vi "Parse Tree Labels.vi"(5 "FIFO Idx Qs":T1, 6 "Channel handle in":u32, 7 "Access":T2, 8 "error out":errorcluster, 10 "Label Refs":T3[](array[typedef]) format="%.0x", 11 "Custom Device Ref":T3 format="%.0x") -> (0 "error out":errorcluster, 1 "Transfer Periods":u32[](array[numeric]), 2 "Label Map":i32[](array[numeric]), 3 "Label data":T4[](array[typedef]) {"Words"."Param Setting"."Num Bits" min=1 max=32; "Words"."Param Setting"."Start Bit" min=8 max=31; "Words"."Block Data Refs"."Data Reference" format="%.0x"; "Label" format="%.0o"})   [LabVIEW 2012, in "AIT 429 Engine.lvlib"]
uses:
  AIT 429 Engine.lvlib
  <vilib>/NI Veristand/Custom Device API/Custom Device Item Ref.ctl
  RT Controls/RT Label Settings.ctl
  Shared/Controls and Global/Label.ctl
  Shared/Controls and Global/transferPeriod.ctl
  RT Controls/Driver Data.ctl
  RT Controls/RT Word Settings.ctl
  <vilib>/NI Veristand/Custom Device API/Block Data Reference.ctl
  <vilib>/NI Veristand/Custom Device API/Data Reference.ctl
  RT Controls/RT Param Setting.ctl
  Shared/Controls and Global/Start Bit.ctl
  Shared/Controls and Global/Number of Bits.ctl
  Shared/Controls and Global/TransferType.ctl
  <vilib>/NI Veristand/Custom Device API/Data Access Type.ctl
  RT Controls/FIFO Idx Qs.ctl
  RT Controls/Data Ref FGV Command.ctl
  Shared/Controls and Global/Global.vi
  <vilib>/NI Veristand/Custom Device Tools/Custom Device Utility Library/NI VeriStand - Search for All Items by GUID.vi
  <vilib>/NI Veristand/Custom Device Tools/Custom Device Utility Library/NI VeriStand - Search for Item by GUID.vi
  <vilib>/NI Veristand/Custom Device API/Get Item Property (U16).vi
  <vilib>/NI Veristand/Custom Device API/Get Item Property (U32).vi
  <vilib>/NI Veristand/Custom Device API/Get Item Property (String).vi
  <vilib>/NI Veristand/Custom Device API/Get Item Property (Boolean).vi
  <vilib>/NI Veristand/Custom Device API/Get Item Property (Double).vi
  <vilib>/NI Veristand/Custom Device API/Get Item Property (I32).vi
  ARINC 429 Shared.lvlib
  <vilib>/NI Veristand/Custom Device API/Custom Device API.lvlib
  <vilib>/NI Veristand/Custom Device Tools/Custom Device Utility Library/Custom Device Utility Library.lvlib
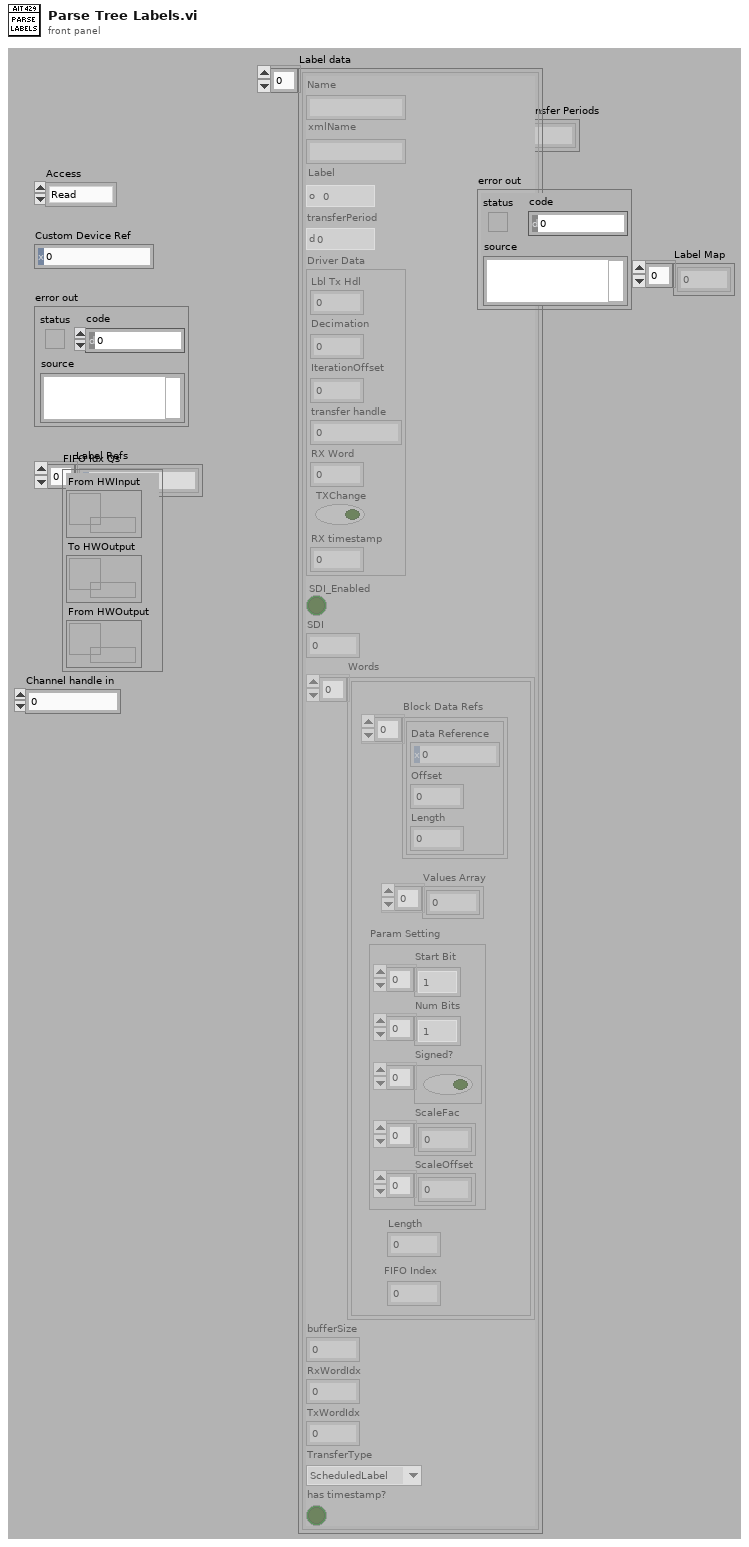
[diagram p1: front panel]
types:
  T1 = typedef "AIT 429 Engine.lvlib/FIFO Idx Qs.ctl" = cluster{"From HWInput":refnum<queue>, "To HWOutput":refnum<queue>, "From HWOutput":refnum<queue>}
  T2 = typedef "Custom Device API.lvlib/Data Access Type.ctl" = enum16{"Read", "Write"}
  T3 = typedef "Custom Device API.lvlib/Custom Device Item Ref.ctl" = u64
  T4 = typedef "AIT 429 Engine.lvlib/RT Label Settings.ctl" = cluster{"Name":string, "xmlName":string, "Label":T5, "transferPeriod":T6, "Driver Data":T7, "SDI_Enabled":bool, "SDI":u8, "Words":T8[], "bufferSize":u32, "RxWordIdx":i32, "TxWordIdx":i32, "TransferType":T14, "has timestamp?":bool}
  T5 = typedef "ARINC 429 Shared.lvlib/Label.ctl" = u8
  T6 = typedef "ARINC 429 Shared.lvlib/transferPeriod.ctl" = u32
  T7 = typedef "AIT 429 Engine.lvlib/Driver Data.ctl" = cluster{"Lbl Tx Hdl":u32, "Decimation":i32, "IterationOffset":i32, "transfer handle":u32, "RX Word":u32, "TXChange":bool, "RX timestamp":dbl}
  T8 = typedef "AIT 429 Engine.lvlib/RT Word Settings.ctl" = cluster{"Block Data Refs":T9[], "Values Array":dbl[], "Length":i32, "FIFO Index":i32, "Param Setting":T11}
  T9 = typedef "Custom Device API.lvlib/Block Data Reference.ctl" = cluster{"Data Reference":T10, "Offset":i32, "Length":i32}
  T10 = typedef "Custom Device API.lvlib/Data Reference.ctl" = i32
  T11 = typedef "AIT 429 Engine.lvlib/RT Param Setting.ctl" = cluster{"Start Bit":T12[], "Num Bits":T13[], "Signed?":bool[], "ScaleFac":dbl[], "ScaleOffset":dbl[]}
  T12 = typedef "ARINC 429 Shared.lvlib/Start Bit.ctl" = i32
  T13 = typedef "ARINC 429 Shared.lvlib/Number of Bits.ctl" = i32
  T14 = typedef "ARINC 429 Shared.lvlib/TransferType.ctl" = enum16{"ScheduledLabel", "Acyclic", "Block", "Strobe"}
  T15 = typedef "AIT 429 Engine.lvlib/Data Ref FGV Command.ctl" = enum16{"Intialize", "Get", "Update"}
  T16 = typedef "Custom Device API.lvlib/Custom Device Item Info.ctl" = cluster{"Name":string, "Is Channel":bool, "GUID":string, "Is Waveform":bool}
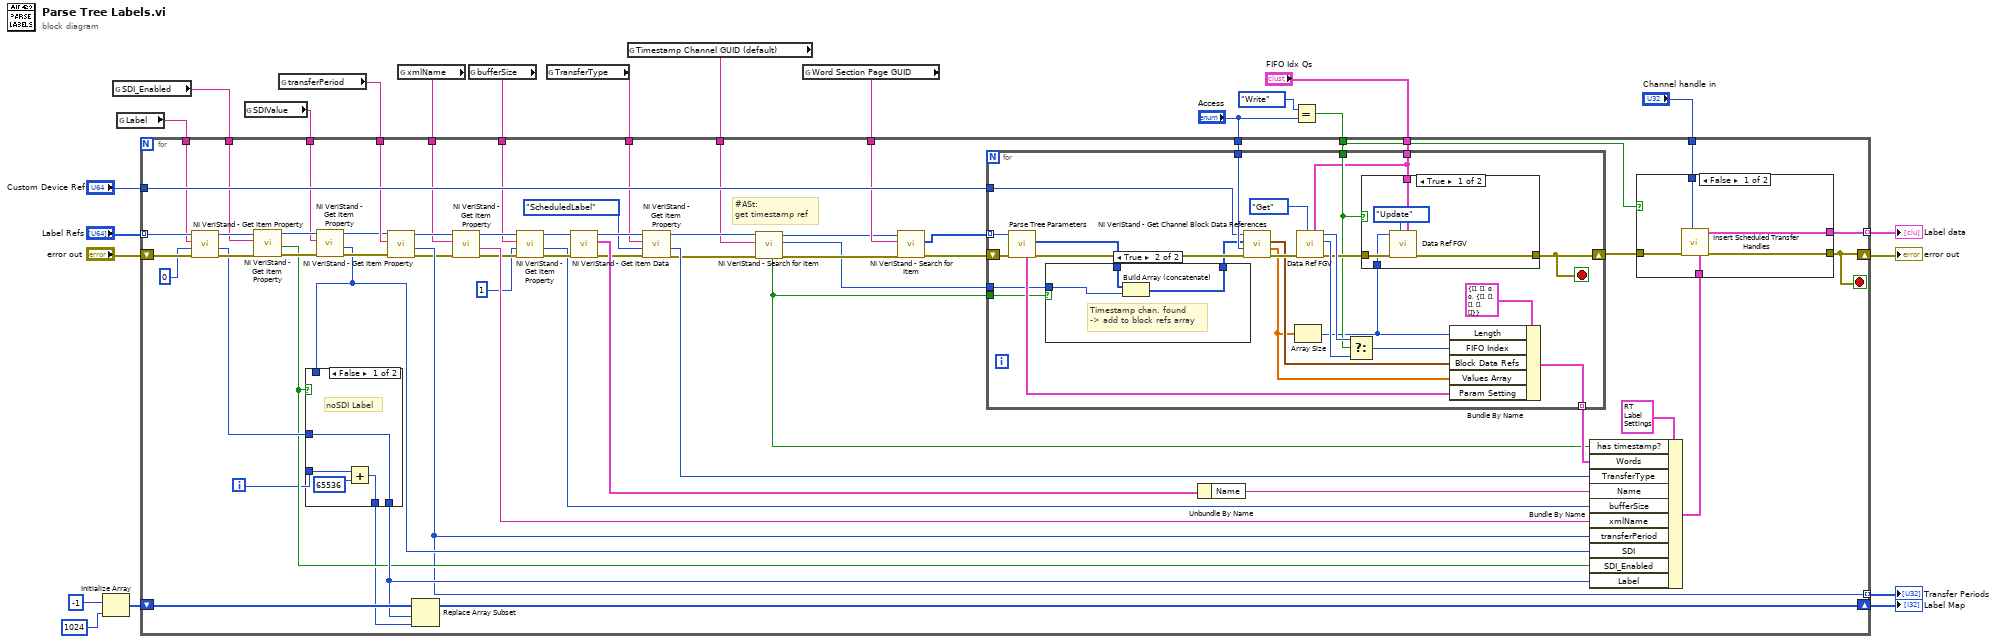
[diagram p0: block diagram]
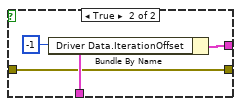
[diagram p2: hidden frame]
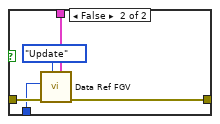
[diagram p4: hidden frame]
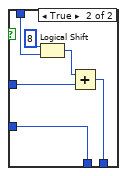
[diagram p5: hidden frame]
diagram:
  n1 = Initialize Array(-1 ("index"), 1024 ("dimension size")) -> (w14:i32[])
  n2 = global read "Global.vi" "SDI_Enabled"() -> (w8:string)
  n3 = global read "Global.vi" "Label"() -> (w12:string)
  n4 = global read "Global.vi" "SDIValue"() -> (w7:string)
  n5 = global read "Global.vi" "transferPeriod"() -> (w11:string)
  n6 = global read "Global.vi" "xmlName"() -> (w6:string)
  n7 = global read "Global.vi" "bufferSize"() -> (w5:string)
  n8 = global read "Global.vi" "TransferType"() -> (w2:string)
  n9 = global read "Global.vi" "Timestamp Channel GUID (default)"() -> (w1:string)
  n10 = global read "Global.vi" "Word Section Page GUID"() -> (w4:string)
  n11 = Equal?(x=Data_Access_Type."Write" ("y"), y="Access") -> (x = y?=w10:bool)
  n12 = for {
    tunnel: "Label Refs" -> [w85] mode=indexing
    shift-right: [w40] -> w20
    shift-left: "error out" -> [w81]
    tunnel: "Access" -> [w82]
    tunnel: "Custom Device Ref" -> [w77]
    tunnel: [w61] -> w24 mode=indexing
    tunnel: "FIFO Idx Qs" -> [w74]
    shift-right: [w78] -> w13
    shift-left: w14 -> [w79]
    tunnel: w12 -> [w76]
    tunnel: w11 -> [w75]
    tunnel: w10 -> [w45]
    tunnel: "Channel handle in" -> [w43]
    tunnel: w8 -> [w71]
    tunnel: w7 -> [w66]
    tunnel: w6 -> [w58]
    tunnel: w5 -> [w51]
    tunnel: w4 -> [w47]
    tunnel: [w41] -> w3 mode=indexing
    tunnel: w2 -> [w35]
    tunnel: w1 -> [w27]
    i -> [w56]
    stop <- w40 stop-if-true
    # "#ASt:\nget timestamp ref"
    n13 = call-poly <vilib>:"NI VeriStand - Get Item Property.vi"("error in (no error)"=w81, "Default Value"=T5 0 ("Label"), "Property Name"=w76, "Item Ref in"=w85) -> ("error out"=w72:errorcluster, "Value"=w65:u32, "Item Ref out"=w73:T3)  [unwired: 4 in, 1 out]
    n14 = call-poly <vilib>:"NI VeriStand - Get Item Property.vi"("error in (no error)"=w72, "Property Name"=w71, "Item Ref in"=w73) -> ("error out"=w68:errorcluster, "Value"=w63:bool, "Item Ref out"=w70:T3)  [unwired: 5 in, 1 out]
    n15 = call-poly <vilib>:"NI VeriStand - Get Item Property.vi"("error in (no error)"=w68, "Property Name"=w66, "Item Ref in"=w70) -> ("error out"=w67:errorcluster, "Value"=w62:u32, "Item Ref out"=w69:T3)  [unwired: 5 in, 1 out]
    n16 = case shown="False" w63 {
      tunnel: w62 -> [_ w142]
      tunnel: w65 -> [w136 w139]
      tunnel: [w136 w138] -> w64
      tunnel: w56 -> [w135 w137]
      tunnel: [w134 w137] -> w55
      frame False {
        # "noSDI Label"
        n17 = Add(x=w135, y=65536) -> (x+y=w134:i32)
      }
      frame True {
        n18 = Logical Shift(y=u32 8 ("x"), x=w142) -> (x << y=w140:u32)
        n19 = Add(x=w140, y=w139) -> (x+y=w138:u32)
      }
    }
    n20 = call-poly <vilib>:"NI VeriStand - Get Item Property.vi"("error in (no error)"=w67, "Property Name"=w75, "Item Ref in"=w69) -> ("error out"=w59:errorcluster, "Value"=w61:u32, "Item Ref out"=w60:T3)  [unwired: 5 in, 1 out]
    n21 = Replace Array Subset(array=w79, new element=w55, index=w64) -> (w78:i32[])
    n22 = call-poly <vilib>:"NI VeriStand - Get Item Property.vi"("error in (no error)"=w59, "Property Name"=w58, "Item Ref in"=w60) -> ("error out"=w54:errorcluster, "Value"=w57:string, "Item Ref out"=w52:T3)  [unwired: 5 in, 1 out]
    n23 = call-poly <vilib>:"NI VeriStand - Get Item Property.vi"("error in (no error)"=w54, "Default Value"=u32 1, "Property Name"=w51, "Item Ref in"=w52) -> ("error out"=w53:errorcluster, "Value"=w50:u32, "Item Ref out"=w49:T3)  [unwired: 4 in, 1 out]
    n24 = call <vilib>:"NI VeriStand - Get Item Data.vi"("error in (no error)"=w53, "Item Ref in"=w49) -> ("error out"=w36:errorcluster, "Item Info"=w83:T16, "Item Ref out"=w37:T3)  [unwired: 6 in, 1 out]
    n25 = call-poly <vilib>:"NI VeriStand - Get Item Property.vi"("error in (no error)"=w36, "Default Value"=TransferType."ScheduledLabel" ("TransferType"), "Property Name"=w35, "Item Ref in"=w37) -> ("error out"=w30:errorcluster, "Value"=w34:u16, "Item Ref out"=w31:T3)  [unwired: 4 in, 1 out]
    n26 = call-poly <vilib>:"NI VeriStand - Search for Item.vi"("error in"=w30, "Item GUID"=w27, "Section Ref in"=w31) -> ("error out"=w29:errorcluster, "Item Ref"=w26:T3, "Section Ref out"=w28:T3, "Found"=w25:bool)  [unwired: 5 in]
    n27 = call-poly <vilib>:"NI VeriStand - Search for Item.vi"("error in"=w29, "Item GUID"=w47, "Section Ref in"=w28) -> ("error out"=w48:errorcluster, "Item Refs"=w39:T3[])  [unwired: 5 in, 2 out]
    n28 = for {
      tunnel: w82 -> [w118]
      tunnel: w77 -> [w111]
      tunnel: w45 -> [w110]
      tunnel: w74 -> [w109]
      shift-right: [w107] -> w42
      shift-left: w48 -> [w108]
      tunnel: w39 -> [w106] mode=indexing
      tunnel: [w101] -> w46 mode=indexing
      tunnel: w25 -> [w97]
      tunnel: w26 -> [w98]
      stop <- w107 stop-if-true
      n29 = call "Parse Tree Parameters.vi"("error in"=w108, "Item Ref in"=w106) -> ("error out"=w117:errorcluster, "Parameter References"=w96:T3[], "Parameter Driver Data"=w104:T11)  [unwired: 6 in, 1 out]
      n30 = case shown="True" w97 {
        tunnel: w98 -> [_ w120]
        tunnel: w96 -> [w119 w122]
        tunnel: [w119 w121] -> w95
        frame False {
        }
        frame True {
          # "Timestamp chan. found\n-> add to block refs array"
          n31 = Build Array (concatenate)(w122, w120) -> (w121:T3[])
        }
      }
      n32 = call <vilib>:"NI VeriStand - Get Channel Block Data References.vi"("error in (no error)"=w117, "Access"=w118, "Channel Refs"=w95, "Device Ref in"=w111) -> ("error out"=w116:errorcluster, "Values Array"=w99:dbl[], "Block Data Refs"=w100:T9[])  [unwired: 4 in, 1 out]
      n33 = Array Size(array=w99) -> (size(s)=w102:i32)
      n34 = call "Data Ref FGV.vi"("FIFO Idx Qs"=w109, "Command"=Data_Ref_FGV_Command."Get", "error in (no error)"=w116) -> ("error out"=w112:errorcluster, "To HWOutput FIFO Index / Length"=w113:i32, "From HWInput FIFO Index / Length"=w114:i32)  [unwired: 5 in, 1 out]
      n35 = Select(t=w114, s=w110, f=w113) -> (s? t:f=w103:i32)
      n36 = case shown="True" w110 {
        tunnel: w112 -> [w127 w132]
        tunnel: [w124 w128] -> w107
        tunnel: w102 -> [w125 w130]
        tunnel: w109 -> [w123 w129]
        frame True {
          n37 = call "Data Ref FGV.vi"("FIFO Idx Qs"=w123, "Command"=Data_Ref_FGV_Command."Update", "error in (no error)"=w127, "From HWInput Length"=w125) -> ("error out"=w124:errorcluster)  [unwired: 4 in, 3 out]
        }
        frame False {
          n38 = call "Data Ref FGV.vi"("FIFO Idx Qs"=w129, "Command"=Data_Ref_FGV_Command."Update", "error in (no error)"=w132, "To HWOutput Length"=w130) -> ("error out"=w128:errorcluster)  [unwired: 4 in, 3 out]
        }
      }
      n39 = Bundle By Name(cluster=T8 {"Block Data Refs"=[], "Values Array"=[], "Length"=0, "FIFO Index"=0, "Param Setting"={"Start Bit"=[], "Num Bits"=[], "Signed?"=[], "ScaleFac"=[], "ScaleOffset"=[]}} ("Word"), "Length"=w102, "FIFO Index"=w103, "Block Data Refs"=w100, "Values Array"=w99, "Param Setting"=w104) -> (w101:T8)
    }
    n40 = Unbundle By Name(w83) -> ("Name"=w38:string)
    n41 = Bundle By Name(cluster=T4 {"Name"="", "xmlName"="", "Label"=0, "transferPeriod"=0, "Driver Data"={"Lbl Tx Hdl"=0, "Decimation"=0, "IterationOffset"=0, "transfer handle"=0, "RX Word"=0, "TXChange"=FALSE, "RX timestamp"=0.0}, "SDI_Enabled"=FALSE, "SDI"=0, "Words"=[], "bufferSize"=0, "RxWordIdx"=0, "TxWordIdx"=0, "TransferType"=enum."ScheduledLabel", "has timestamp?"=FALSE} ("Label"), "has timestamp?"=w25, "Words"=w46, "TransferType"=w34, "Name"=w38, "bufferSize"=w50, "xmlName"=w57, "transferPeriod"=w61, "SDI"=w62, "SDI_Enabled"=w63, "Label"=w64) -> (w44:T4)
    n42 = case shown="False" w45 {
      tunnel: w44 -> [w89 w94]
      tunnel: w43 -> [w90 _]
      tunnel: w42 -> [w88 w92]
      tunnel: [w87 w92] -> w40
      tunnel: [w86 w91] -> w41
      frame False {
        n43 = call "Insert Scheduled Transfer Handles.vi"("Label in"=w89, "Tx channel handle in"=w90, "error in (no error)"=w88) -> ("error out"=w87:errorcluster, "Label out"=w86:T4)  [unwired: 7 in]
      }
      frame True {
        n44 = Bundle By Name(cluster=w94, "Driver Data.IterationOffset"=-1) -> (w91:T4)
      }
    }
  }
  "Transfer Periods" <- w24
  "Label data" <- w3
  "error out" <- w20
  "Label Map" <- w13
